vi "Configure Tx Parameters.vi"(8 "error in":errorcluster, 9 "Radio1 Configuration":T1={"Ch1 Rx Frequency"=2000000000.0, "Ch1 Tx Frequency"=2000000000.0, "Ch1 Rx Gain"=0.0, "Ch1 Tx Gain"=0.0} {"Ch1 Tx Frequency" format="%#_6p"; "Ch1 Rx Frequency" format="%#_6p"}, 10 "Radio0 Configuration":T2={"Ch0 Rx Frequency"=2000000000.0, "Ch0 Tx Frequency"=2000000000.0, "Ch0 Rx Gain"=0.0, "Ch0 Tx Gain"=0.0} {"Ch0 Tx Frequency" format="%#_6p"; "Ch0 Rx Frequency" format="%#_6p"}, 11 "session In":T4) -> (0 "error out":errorcluster, 3 "session out":T3)   [LabVIEW 2023]
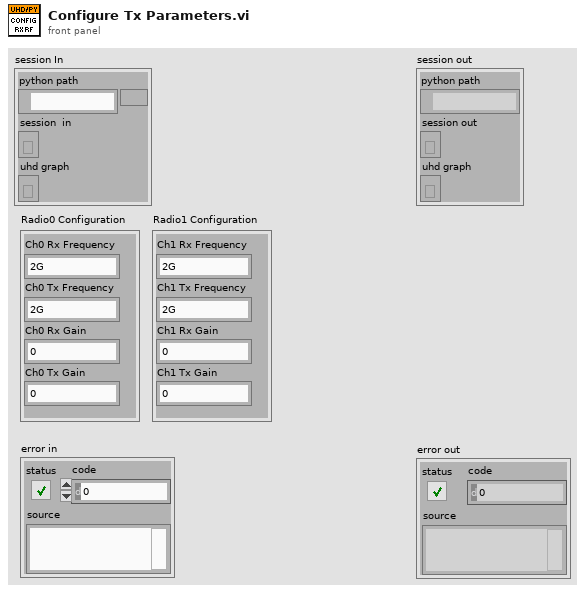
[diagram p1: front panel]
types:
  T1 = cluster{"Ch1 Rx Frequency":dbl, "Ch1 Tx Frequency":dbl, "Ch1 Rx Gain":dbl, "Ch1 Tx Gain":dbl}
  T2 = cluster{"Ch0 Rx Frequency":dbl, "Ch0 Tx Frequency":dbl, "Ch0 Rx Gain":dbl, "Ch0 Tx Gain":dbl}
  T3 = cluster{"python path":path, "session out ":refnum<k35>, "uhd graph":refnum<k38>}
  T4 = cluster{"python path":path, "session  in":refnum<k35>, "uhd graph":refnum<k38>}
  T5 = cluster{"python path":path, "session out":refnum<k35>, "uhd graph":refnum<k38>}
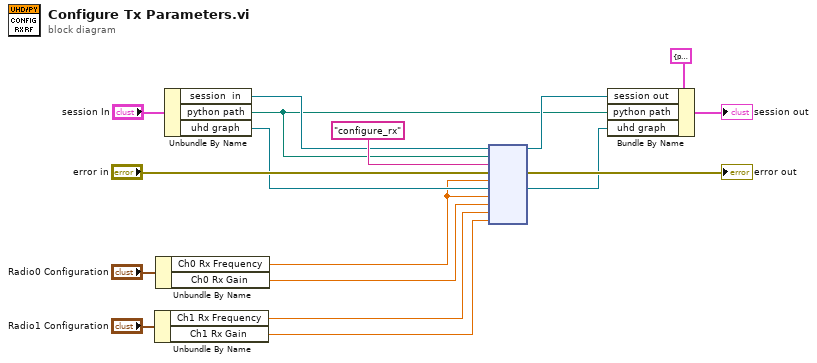
[diagram p0: block diagram]
diagram:
  n1 = Unbundle By Name("Radio1 Configuration") -> ("Ch1 Rx Frequency"=w2:dbl, "Ch1 Rx Gain"=w1:dbl)
  n2 = Unbundle By Name("Radio0 Configuration") -> ("Ch0 Rx Frequency"=w4:dbl, "Ch0 Rx Gain"=w3:dbl)
  n3 = Unbundle By Name("session In") -> ("session  in"=w13:refnum<k35>, "python path"=w9:path, "uhd graph"=w14:refnum<k38>)
  n4 = node(w13, w9, "configure_rx" ("function name"), "error in", w4, w14, w4, w3, w2, w1) -> (w11:refnum<k35>, →"error out":errorcluster, w10:refnum<k38>)  [unwired: 5 in, 2 out]
  n5 = Bundle By Name(cluster=T5 {"python path"=path "", "session out"=refnum, "uhd graph"=refnum}, "session out"=w11, "python path"=w9, "uhd graph"=w10) -> (→"session out":T5)
